vi "1C.1 Camera - FindStern.vi"(11 "Refnum in":T3) -> (0 "Stern Found":T1, 1 "y pixel":i32, 2 "x pixel":i32, 3 "Refnum out":T3(plugin-control), 4 "Heading":T2 format="%05.1f")   [LabVIEW 2011]
uses:
  <vilib>/vision/Image Controls.llb/IMAQ Image.ctl
  2-RIO/2 Typedefs/heading.ctl
  2-RIO/2 Typedefs/indicator LED.ctl
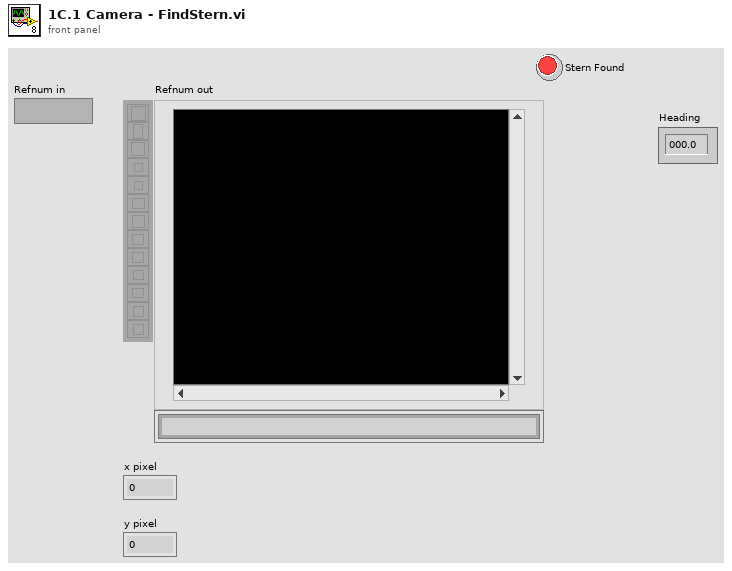
[diagram p1: front panel]
types:
  T1 = typedef "indicator LED.ctl" = bool
  T2 = typedef "heading.ctl" = dbl
  T3 = typedef "IMAQ Image.ctl" = refnum<image>
  T4 = cluster{"Position":cluster{"x":sgl, "y":sgl}, "Angle":sgl, "Scale":sgl, "Score":sgl, "Bounding Box":cluster{"x":sgl, "y":sgl}[]}[]
  T5 = cluster{"Position":cluster{"x":sgl, "y":sgl}, "Angle":sgl, "Scale":sgl, "Score":sgl, "Bounding Box":cluster{"x":sgl, "y":sgl}[]}
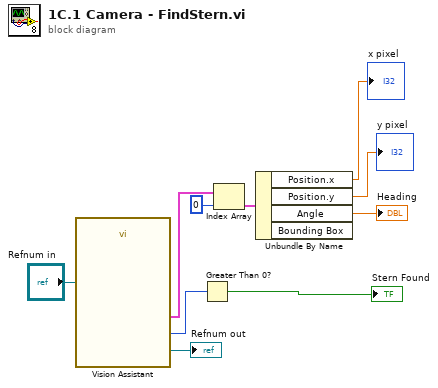
[diagram p0: block diagram]
diagram:
  n1 = call "Vision Assistant"("Image In"="Refnum in") -> ("Image Out"=→"Refnum out":T3, "Matches (Color Pattern Matching 1)"=w7:T4, "Number of Matches (Color Pattern Matching 1)"=w3:i32)  [unwired: 23 in, 1 out]
  n2 = Greater Than 0?(x=w3) -> (x > 0?=→"Stern Found":bool)
  n3 = Index Array(array=w7, index=0) -> (element=w6:T5)
  n4 = Unbundle By Name(w6) -> ("Position.x"=→"x pixel":sgl, "Position.y"=→"y pixel":sgl, "Angle"=→"Heading":sgl)  [unwired: 1 out]
